vi "Disabled.vi"(7 "Robot Mode":T2, 10 "Match Info":T1={"Autonomous Elapsed Seconds"=0.0, "TeleOp Elapsed Seconds"=0.0, "Disabled Elapsed Seconds"=0.0, "Visited Autonomous"=FALSE, "Visited TeleOp"=FALSE, "Visited Disabled"=FALSE, "Autonomous Settings"={"Autonomous Style"=enum."Independent", "VI Refnum"=refnum}}, 11 "Call Context":T3) -> ()   [LabVIEW 2017]
doc: "This VI is called each time a disabled packet is received from the DS. It is often used to prepare for the next robot mode, to calibrate sensors, etc."
uses:
  <vilib>/Rock Robotics/WPI/DriverStation/WPI_DriverStationDerivedRobotMode.ctl
  <vilib>/Rock Robotics/WPI/DriverStation/WPI_DriverStationRobotMode2.ctl
  <vilib>/Rock Robotics/WPI/DriverStation/WPI_DriverStationMatch Info.ctl
  LEDs/LED Notifier.ctl
  LEDs/LED Control Type.ctl
  <vilib>/Rock Robotics/Network Tables/NT Read Boolean.vi
  LEDs/LED Globals.vi
  <vilib>/Rock Robotics/Network Tables/NT Write String.vi
  <vilib>/Rock Robotics/Network Tables/NT Read String.vi
  Drive/Drive Globals.vi
  Intake Rotation/Intake Rotation Globals.vi
  Lift/Lift Globals.vi
  RPED/RPED Globals.vi
  Autonomous/Autonomous Globals.vi
panel:
  out "error out":errorcluster
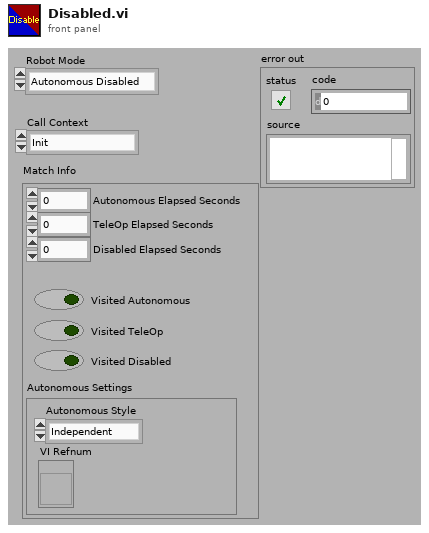
[diagram p1: front panel]
types:
  T1 = typedef "WPI_DriverStationMatch Info.ctl" = cluster{"Autonomous Elapsed Seconds":dbl, "TeleOp Elapsed Seconds":dbl, "Disabled Elapsed Seconds":dbl, "Visited Autonomous":bool, "Visited TeleOp":bool, "Visited Disabled":bool, "Autonomous Settings":cluster{"Autonomous Style":enum16{"Iterative", "Independent"}, "VI Refnum":refnum<vi>}}
  T2 = typedef "WPI_DriverStationRobotMode2.ctl" = enum16{"Autonomous Disabled", "Autonomous Enabled", "Teleop Disabled", "Teleop Enabled", "Disconnected", "Finish", "Test Disabled", "Test Enabled", "Emergency Stopped"}
  T3 = typedef "WPI_DriverStationDerivedRobotMode.ctl" = enum16{"Init", "Execute", "Stop"}
  T4 = typedef "LED Notifier.ctl" = cluster{"LED Control Type":T5, "Climbing":bool, "Auto Tracking":bool, "Ready for Cube Floor":bool, "Ready for Cube Portal":bool}
  T5 = typedef "LED Control Type.ctl" = enum16{"Off", "Waiting On Field", "Connected ", "Cube In Intake", "Climbing", "Auto Cube Capture", "Ready for Cube Floor", "Ready for Cube Portal"}
  T6 = enum16{"open", "replace", "create", "open or create", "replace or create", "replace or create with confirmation"}
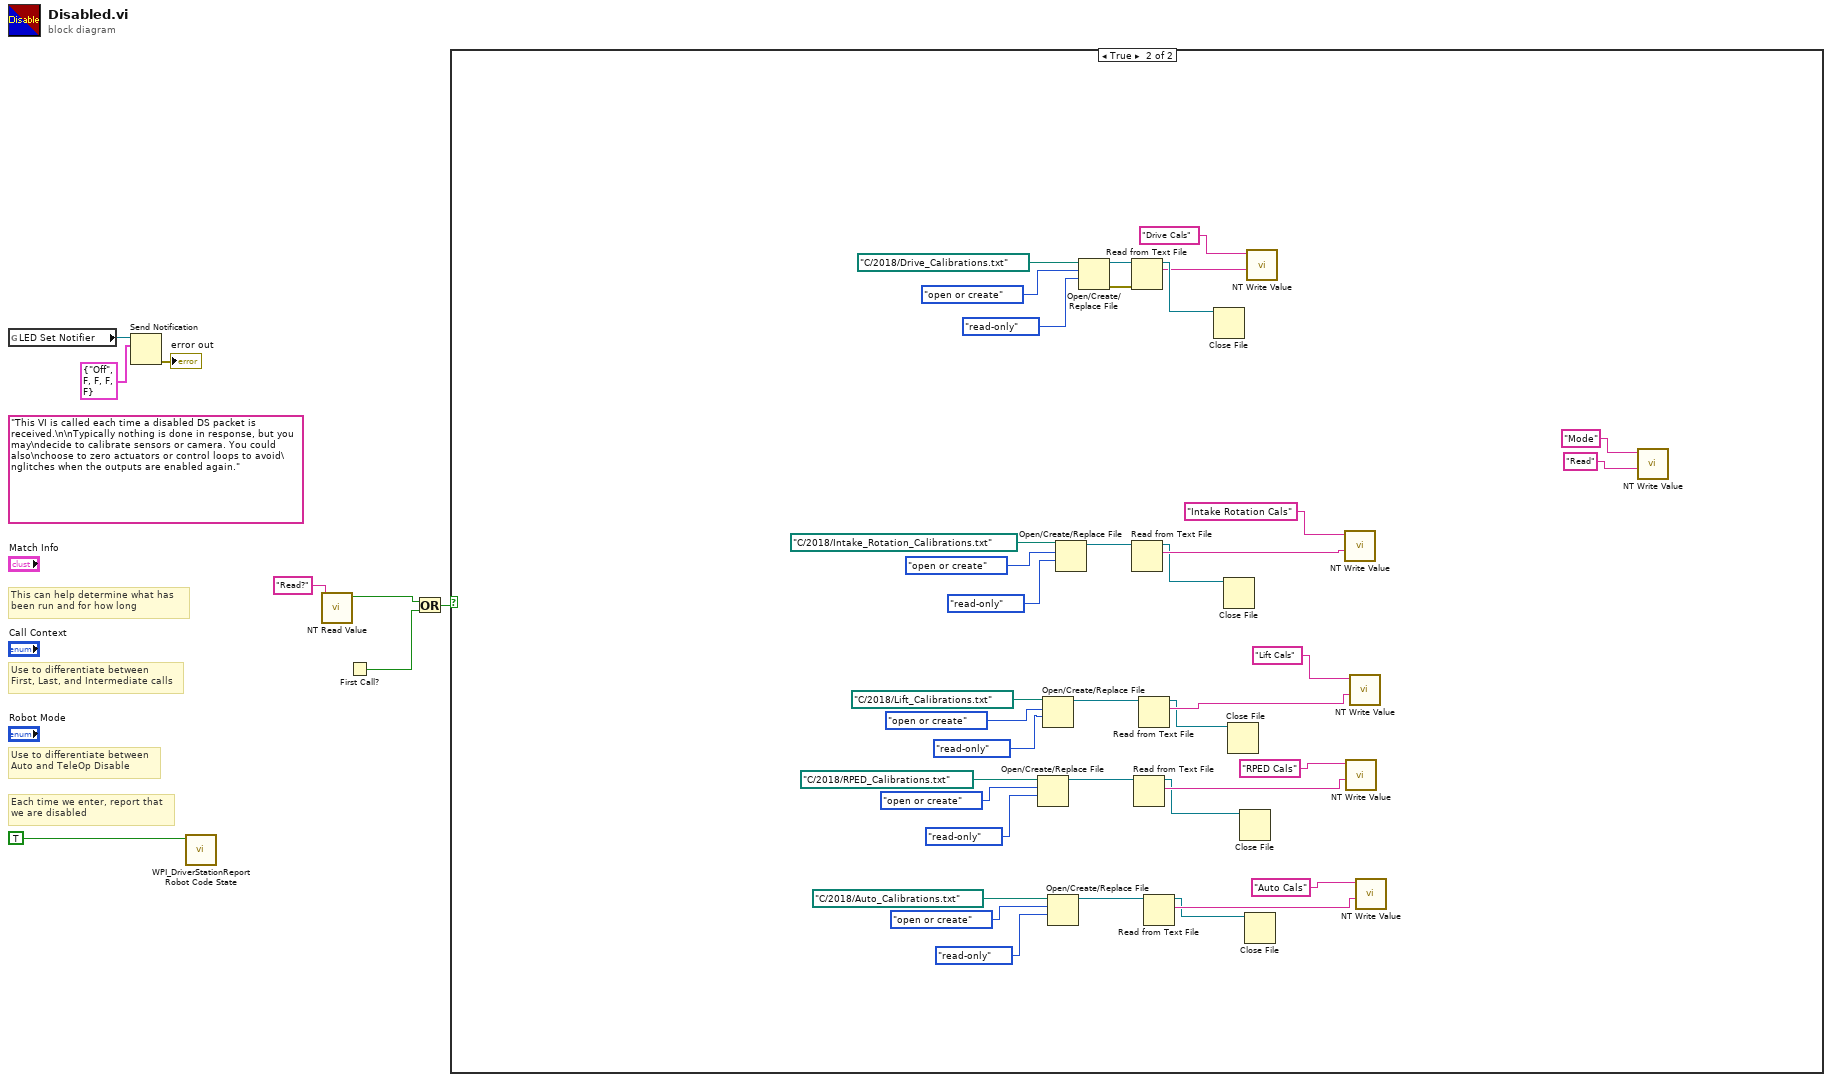
[diagram p0: block diagram]
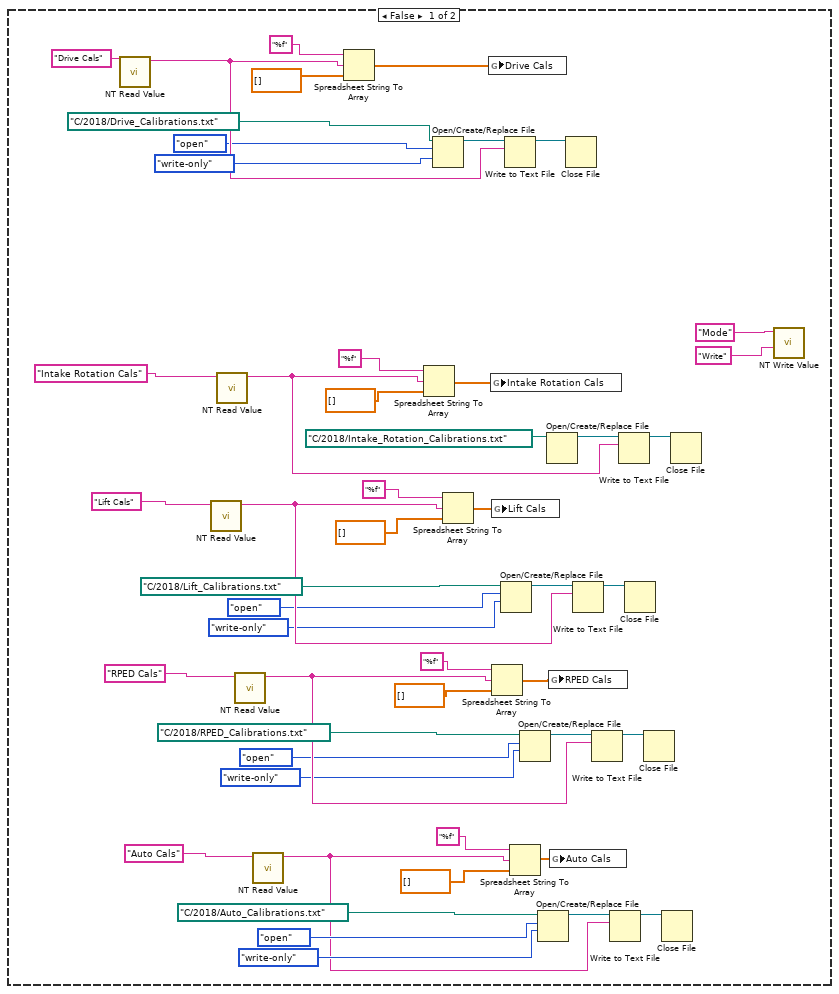
[diagram p2: hidden frame]
diagram:
  (unwired) "This VI is called each time a disabled DS packet is received.\n\nTypically nothing is done in response, but you may\ndecide to calibrate sensors or camera. You could also\nchoose to zero actuators or control loops to avoid\nglitches when the outputs are enabled again."
  # "Each time we enter, report that\nwe are disabled"
  # "Use to differentiate between\nFirst, Last, and Intermediate calls"
  # "This can help determine what has\nbeen run and for how long"
  # "Use to differentiate between\nAuto and TeleOp Disable"
  n1 = global read "LED Globals.vi" "LED Set Notifier"() -> (w7:refnum<notifier>)
  n2 = Send Notification(notification=T4 {"LED Control Type"=enum."Off", "Climbing"=FALSE, "Auto Tracking"=FALSE, "Ready for Cube Floor"=FALSE, "Ready for Cube Portal"=FALSE} ("LED Notifier"), notifier=w7) -> (error out=→"error out":errorcluster)  [unwired: 1 in, 1 out]
  n3 = call <vilib>:"WPI_DriverStationReport Robot Code State.vi"("Disabled"=TRUE ("Autonomous")) -> ()  [unwired: 10 in, 1 out]
  n4 = call-poly <vilib>:"NT Read Value.vi"("Name"="Read?") -> ("Boolean"=w2:bool)  [unwired: 9 in, 1 out]
  n5 = First Call?() -> (First Call?: T/F=w1:bool)
  n6 = Or(x=w2, y=w1) -> (x .or. y?=w3:bool)
  n7 = case shown="True" w3 {
    frame False {
      n8 = call-poly <vilib>:"NT Read Value.vi"("Name"="Drive Cals") -> ("String"=w47:string)  [unwired: 9 in, 1 out]
      n9 = call-poly <vilib>:"NT Read Value.vi"("Name"="Lift Cals") -> ("String"=w35:string)  [unwired: 9 in, 1 out]
      n10 = call-poly <vilib>:"NT Read Value.vi"("Name"="Intake Rotation Cals") -> ("String"=w41:string)  [unwired: 9 in, 1 out]
      n11 = call-poly <vilib>:"NT Read Value.vi"("Name"="RPED Cals") -> ("String"=w29:string)  [unwired: 9 in, 1 out]
      n12 = call-poly <vilib>:"NT Read Value.vi"("Name"="Auto Cals") -> ("String"=w16:string)  [unwired: 9 in, 1 out]
      n13 = Spreadsheet String To Array(format string="%f", spreadsheet string=w47, array type (2D Dbl)=dbl[] []) -> (array=w19:dbl[])  [unwired: 1 in]
      n14 = Spreadsheet String To Array(format string="%f", spreadsheet string=w41, array type (2D Dbl)=dbl[] []) -> (array=w22:dbl[])  [unwired: 1 in]
      n15 = Open/Create/Replace File(file path (use dialog)=path "C:/2018/Drive_Calibrations.txt" ("file (use dialog)"), operation (0:open)=T6."open", access (0:read/write)=enum16{"read/write", "read-only", "write-only"}."write-only") -> (refnum out=w51:refnum<file>)  [unwired: 3 in, 2 out]
      n16 = Spreadsheet String To Array(format string="%f", spreadsheet string=w35, array type (2D Dbl)=dbl[] []) -> (array=w21:dbl[])  [unwired: 1 in]
      n17 = global write "Drive Globals.vi" "Drive Cals"(w19) -> ()
      n18 = global write "Intake Rotation Globals.vi" "Intake Rotation Cals"(w22) -> ()
      n19 = global write "Lift Globals.vi" "Lift Cals"(w21) -> ()
      n20 = Spreadsheet String To Array(format string="%f", spreadsheet string=w29, array type (2D Dbl)=dbl[] []) -> (array=w20:dbl[])  [unwired: 1 in]
      n21 = Open/Create/Replace File(file path (use dialog)=path "C:/2018/Lift_Calibrations.txt" ("file (use dialog)"), operation (0:open)=T6."open", access (0:read/write)=enum16{"read/write", "read-only", "write-only"}."write-only") -> (refnum out=w37:refnum<file>)  [unwired: 3 in, 2 out]
      n22 = Write to Text File(file (use dialog)=w51, text=w47) -> (refnum out=w52:refnum<file>)  [unwired: 2 in, 2 out]
      n23 = Spreadsheet String To Array(format string="%f", spreadsheet string=w16, array type (2D Dbl)=dbl[] []) -> (array=w9:dbl[])  [unwired: 1 in]
      n24 = Open/Create/Replace File(file path (use dialog)=path "C:/2018/RPED_Calibrations.txt" ("file (use dialog)"), operation (0:open)=T6."open", access (0:read/write)=enum16{"read/write", "read-only", "write-only"}."write-only") -> (refnum out=w31:refnum<file>)  [unwired: 3 in, 2 out]
      n25 = Open/Create/Replace File(file path (use dialog)=path "C:/2018/Auto_Calibrations.txt" ("file (use dialog)"), operation (0:open)=T6."open", access (0:read/write)=enum16{"read/write", "read-only", "write-only"}."write-only") -> (refnum out=w14:refnum<file>)  [unwired: 3 in, 2 out]
      n26 = Open/Create/Replace File(file path (use dialog)=path "C:/2018/Intake_Rotation_Calibrations.txt" ("file (use dialog)")) -> (refnum out=w43:refnum<file>)  [unwired: 5 in, 2 out]
      n27 = global write "RPED Globals.vi" "RPED Cals"(w20) -> ()
      n28 = global write "Autonomous Globals.vi" "Auto Cals"(w9) -> ()
      n29 = Close File(refnum=w52) -> ()  [unwired: 1 in, 2 out]
      n30 = Write to Text File(file (use dialog)=w37, text=w35) -> (refnum out=w38:refnum<file>)  [unwired: 2 in, 2 out]
      n31 = Write to Text File(file (use dialog)=w31, text=w29) -> (refnum out=w32:refnum<file>)  [unwired: 2 in, 2 out]
      n32 = Write to Text File(file (use dialog)=w14, text=w16) -> (refnum out=w13:refnum<file>)  [unwired: 2 in, 2 out]
      n33 = Write to Text File(file (use dialog)=w43, text=w41) -> (refnum out=w44:refnum<file>)  [unwired: 2 in, 2 out]
      n34 = Close File(refnum=w38) -> ()  [unwired: 1 in, 2 out]
      n35 = Close File(refnum=w32) -> ()  [unwired: 1 in, 2 out]
      n36 = Close File(refnum=w13) -> ()  [unwired: 1 in, 2 out]
      n37 = Close File(refnum=w44) -> ()  [unwired: 1 in, 2 out]
      n38 = call-poly <vilib>:"NT Write Value.vi"("String"="Write", "Name"="Mode") -> ()  [unwired: 9 in, 1 out]
    }
    frame True {
      n39 = Open/Create/Replace File(file path (use dialog)=path "C:/2018/RPED_Calibrations.txt" ("file (use dialog)"), operation (0:open)=T6."open or create", access (0:read/write)=enum16{"read/write", "read-only", "write-only"}."read-only") -> (refnum out=w94:refnum<file>)  [unwired: 3 in, 2 out]
      n40 = Open/Create/Replace File(file path (use dialog)=path "C:/2018/Lift_Calibrations.txt" ("file (use dialog)"), operation (0:open)=T6."open or create", access (0:read/write)=enum16{"read/write", "read-only", "write-only"}."read-only") -> (refnum out=w95:refnum<file>)  [unwired: 3 in, 2 out]
      n41 = Open/Create/Replace File(file path (use dialog)=path "C:/2018/Auto_Calibrations.txt" ("file (use dialog)"), operation (0:open)=T6."open or create", access (0:read/write)=enum16{"read/write", "read-only", "write-only"}."read-only") -> (refnum out=w67:refnum<file>)  [unwired: 3 in, 2 out]
      n42 = Open/Create/Replace File(file path (use dialog)=path "C:/2018/Intake_Rotation_Calibrations.txt" ("file (use dialog)"), operation (0:open)=T6."open or create", access (0:read/write)=enum16{"read/write", "read-only", "write-only"}."read-only") -> (refnum out=w96:refnum<file>)  [unwired: 3 in, 2 out]
      n43 = Open/Create/Replace File(file path (use dialog)=path "C:/2018/Drive_Calibrations.txt" ("file (use dialog)"), operation (0:open)=T6."open or create", access (0:read/write)=enum16{"read/write", "read-only", "write-only"}."read-only") -> (refnum out=w90:refnum<file>, error out=w89:errorcluster)  [unwired: 3 in, 1 out]
      n44 = Read from Text File(file (use dialog)=w90, error in=w89) -> (refnum out=w64:refnum<file>, text=w59:string)  [unwired: 2 in, 2 out]
      n45 = Read from Text File(file (use dialog)=w96) -> (refnum out=w63:refnum<file>, text=w82:string)  [unwired: 3 in, 2 out]
      n46 = Read from Text File(file (use dialog)=w94) -> (refnum out=w61:refnum<file>, text=w78:string)  [unwired: 3 in, 2 out]
      n47 = Read from Text File(file (use dialog)=w95) -> (refnum out=w62:refnum<file>, text=w80:string)  [unwired: 3 in, 2 out]
      n48 = Read from Text File(file (use dialog)=w67) -> (refnum out=w60:refnum<file>, text=w71:string)  [unwired: 3 in, 2 out]
      n49 = Close File(refnum=w64) -> ()  [unwired: 1 in, 2 out]
      n50 = Close File(refnum=w63) -> ()  [unwired: 1 in, 2 out]
      n51 = Close File(refnum=w62) -> ()  [unwired: 1 in, 2 out]
      n52 = Close File(refnum=w61) -> ()  [unwired: 1 in, 2 out]
      n53 = Close File(refnum=w60) -> ()  [unwired: 1 in, 2 out]
      n54 = call-poly <vilib>:"NT Write Value.vi"("String"=w59, "Name"="Drive Cals") -> ()  [unwired: 9 in, 1 out]
      n55 = call-poly <vilib>:"NT Write Value.vi"("String"=w82, "Name"="Intake Rotation Cals") -> ()  [unwired: 9 in, 1 out]
      n56 = call-poly <vilib>:"NT Write Value.vi"("String"=w78, "Name"="RPED Cals") -> ()  [unwired: 9 in, 1 out]
      n57 = call-poly <vilib>:"NT Write Value.vi"("String"=w80, "Name"="Lift Cals") -> ()  [unwired: 9 in, 1 out]
      n58 = call-poly <vilib>:"NT Write Value.vi"("String"=w71, "Name"="Auto Cals") -> ()  [unwired: 9 in, 1 out]
      n59 = call-poly <vilib>:"NT Write Value.vi"("String"="Read", "Name"="Mode") -> ()  [unwired: 9 in, 1 out]
    }
  }
